vi "util_generate_actions.vi"(7 "hmi_references":T2, 8 "error in (no error)":errorcluster) -> (0 "error out":errorcluster, 3 "actions []":cluster{"index":i32, "action":T1}[](array[cluster]))   [LabVIEW 2015, in "lv-build-interface.lvlib"]
uses:
  lv-build-interface.lvlib
  _controls/hmi_references.ctl
  _controls/action.ctl
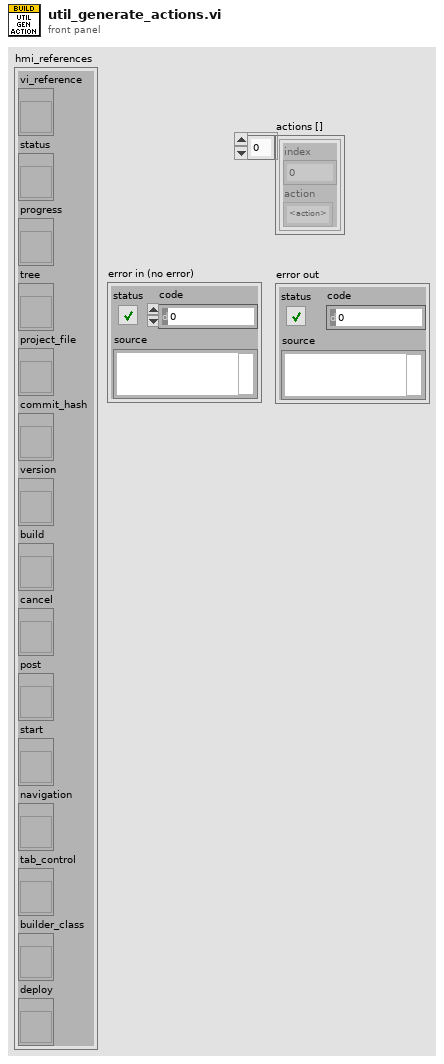
[diagram p1: front panel]
types:
  T1 = typedef "lv-build-interface.lvlib/action.ctl" = enum16{"<action>", "build", "post", "deploy", "<null>"}
  T2 = typedef "lv-build-interface.lvlib/hmi_references.ctl" = cluster{"vi_reference":refnum<vi>, "status":refnum<vi>, "progress":refnum<vi>, "tree":refnum<vi>, "project_file":refnum<vi>, "commit_hash":refnum<vi>, "version":refnum<vi>, "build":refnum<vi>, "cancel":refnum<vi>, "post":refnum<vi>, "start":refnum<vi>, "navigation":refnum<vi>, "tab_control":refnum<vi>, "builder_class":refnum<vi>, "deploy":refnum<vi>}
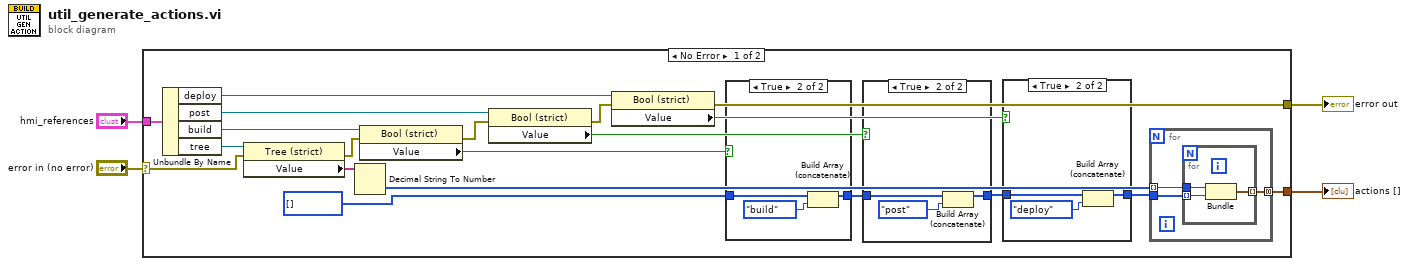
[diagram p0: block diagram]
diagram:
  n1 = case shown="No Error" "error in (no error)" {
    selector: "error in (no error)" -> [w15 w43]
    tunnel: "hmi_references" -> [w24 _]
    tunnel: [w12 _] -> w2
    tunnel: [w8 w43] -> w1
    frame No Error {
      w18 = T1[] [] items=["<action>", "build", "post", "deploy", "<null>"] ("Array")
      n2 = Unbundle By Name(w24) -> ("deploy"=w10:refnum<vi>, "post"=w20:refnum<vi>, "build"=w21:refnum<vi>, "tree"=w16:refnum<vi>)
      n3 = property class="Tree (strict)"(reference=w16, error in=w15) -> (error out=w14:errorcluster, "Value"=w23:string[])  [unwired: 1 out]
      n4 = Decimal String To Number(string=w23) -> (number=w22:i32[])  [unwired: 2 in, 1 out]
      n5 = property class="Bool (strict)"(reference=w21, error in=w14) -> (error out=w19:errorcluster, "Value"=w17:bool)  [unwired: 1 out]
      n6 = property class="Bool (strict)"(reference=w20, error in=w19) -> (error out=w9:errorcluster, "Value"=w11:bool)  [unwired: 1 out]
      n7 = property class="Bool (strict)"(reference=w10, error in=w9) -> (error out=w8:errorcluster, "Value"=w5:bool)  [unwired: 1 out]
      n8 = case shown="True" w17 {
        tunnel: w18 -> [w33 w36]
        tunnel: [w33 w35] -> w13
        frame False {
        }
        frame True {
          n9 = Build Array (concatenate)(w36, action."build" ("action")) -> (w35:T1[])
        }
      }
      n10 = case shown="True" w11 {
        tunnel: w13 -> [w29 w32]
        tunnel: [w29 w31] -> w7
        frame False {
        }
        frame True {
          n11 = Build Array (concatenate)(w32, action."post" ("action")) -> (w31:T1[])
        }
      }
      n12 = case shown="True" w5 {
        tunnel: w7 -> [w25 w28]
        tunnel: [w25 w27] -> w6
        frame False {
        }
        frame True {
          n13 = Build Array (concatenate)(w28, action."deploy" ("action")) -> (w27:T1[])
        }
      }
      n14 = for {
        tunnel: w22 -> [w39] mode=indexing
        tunnel: [w38] -> w12 mode=concatenating
        tunnel: w6 -> [w37]
        n15 = for {
          tunnel: w39 -> [w41]
          tunnel: [w42] -> w38 mode=indexing
          tunnel: w37 -> [w40] mode=indexing
          n16 = Bundle(w41, "action"=w40) -> (w42:cluster{i32, "action":T1})  [unwired: 1 in]
        }
      }
    }
    frame Error {
    }
  }
  "error out" <- w1
  "actions []" <- w2
